vi "checkTimeout.vi"(8 "error in (no error)":errorcluster, 10 "ElectrometerController in":refnum<class "ElectrometerController.lvclass">, 11 "State in":refnum<class "ElectrometerState.lvclass">) -> (0 "error out":errorcluster, 1 "timeout?":bool, 2 "ElectrometerController out":refnum<class "ElectrometerController.lvclass">, 3 "State out":refnum<class "ElectrometerState.lvclass">)   [LabVIEW 2016, in "ElectrometerState.lvclass"]
uses:
  ElectrometerState.lvclass
  ElectrometerController/ElectrometerController.lvclass
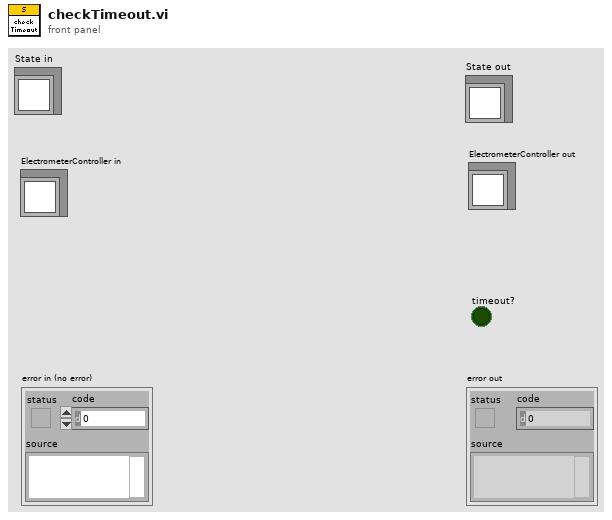
[diagram p1: front panel]
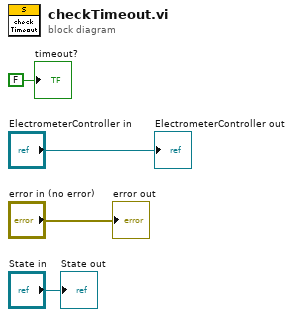
[diagram p0: block diagram]
diagram:
  "error out" <- "error in (no error)"
  "State out" <- "State in"
  "ElectrometerController out" <- "ElectrometerController in"
  "timeout?" <- FALSE ("timeout?")
